vi "Setpoints.vi"(0 "Button 1":bool=TRUE, 5 "Button 2":bool=TRUE, 7 "Button 3":bool=TRUE, 9 "Button 4":bool=TRUE, 11 "Button 5":bool=TRUE) -> ()   [LabVIEW 2014]
uses:
  Robot Global Data.vi
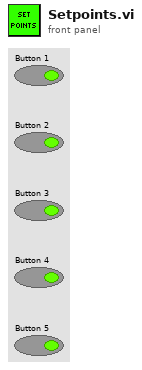
[diagram p1: front panel]
types:
  T1 = enum16{"None", "Bottom Setpoint", "Lower Setpoint", "Mid Setpoint", "Upper Setpoint", "Top Setpoint"}
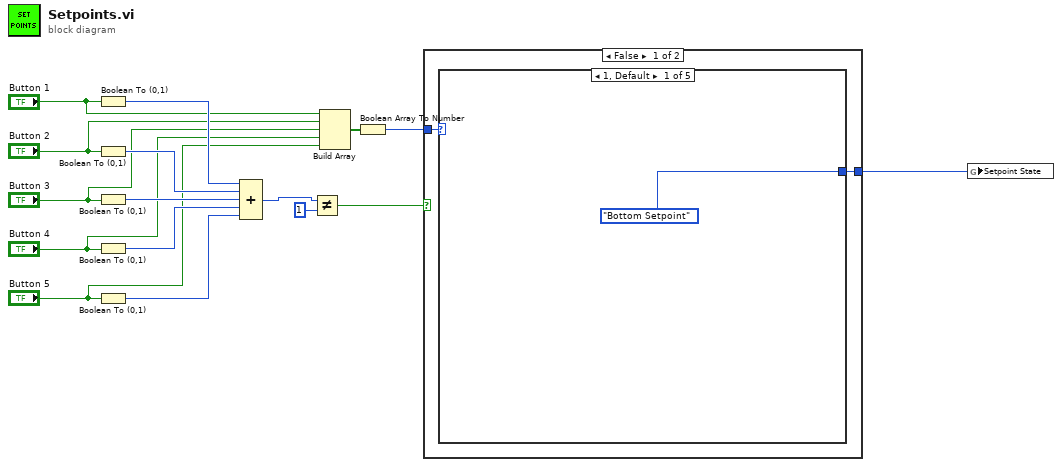
[diagram p0: block diagram]
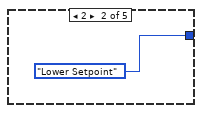
[diagram p2: hidden frame]
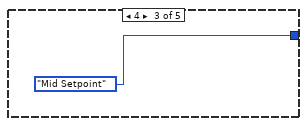
[diagram p3: hidden frame]
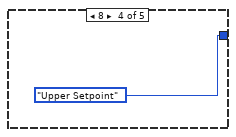
[diagram p4: hidden frame]
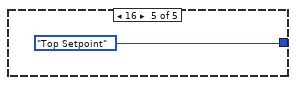
[diagram p5: hidden frame]
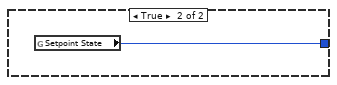
[diagram p6: hidden frame]
diagram:
  n1 = Boolean To (0,1)(Boolean="Button 1") -> (0, 1=w16:i16)
  n2 = Boolean To (0,1)(Boolean="Button 2") -> (0, 1=w15:i16)
  n3 = Boolean To (0,1)(Boolean="Button 3") -> (0, 1=w14:i16)
  n4 = Boolean To (0,1)(Boolean="Button 4") -> (0, 1=w13:i16)
  n5 = Boolean To (0,1)(Boolean="Button 5") -> (0, 1=w12:i16)
  n6 = Compound Arithmetic op=ADD(w16, w15, w14, w13, w12) -> (w1:i16)
  n7 = Not Equal?(x=w1, y=i16 1) -> (x != y?=w2:bool)
  n8 = Build Array("Button 1", "Button 2", "Button 3", "Button 4", "Button 5") -> (w7:bool[])
  n9 = Boolean Array To Number(Boolean array=w7) -> (number=w6:u32)
  n10 = case shown="False" w2 {
    tunnel: w6 -> [w18 _]
    tunnel: [w17 w24] -> w5
    frame False {
      n11 = case shown="1, Default" w18 {
        tunnel: [T1."Bottom Setpoint" ("Setpoint State") T1."Lower Setpoint" ("Setpoint State") T1."Mid Setpoint" ("Setpoint State") T1."Upper Setpoint" ("Setpoint State") T1."Top Setpoint" ("Setpoint State")] -> w17
        frame 1, Default {
        }
        frame 2 {
        }
        frame 4 {
        }
        frame 8 {
        }
        frame 16 {
        }
      }
    }
    frame True {
      n12 = global read "Robot Global Data.vi" "Setpoint State"() -> (w24:T1)
    }
  }
  n13 = global write "Robot Global Data.vi" "Setpoint State"(w5) -> ()
